vi "Configure Basic Sweep.vi"(7 "Timeout (0s)":dbl, 8 "error in (no error)":errorcluster, 9 "Repeat (T: Enable)":bool=TRUE, 10 "Pre Sweep Delay (0s)":dbl, 11 "VISA resource name":refnum<visa-resource-name>) -> (0 "error out":errorcluster, 3 "VISA resource name out":refnum<visa-resource-name>)   [LabVIEW 2014, in "Stanford Research SR1.lvlib"]
doc: "Configures the basic attributes of the Sweep."
uses:
  Stanford Research SR1.lvlib
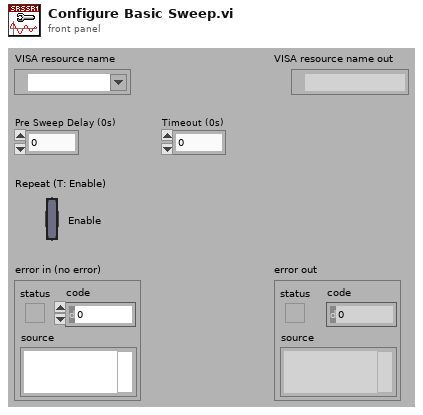
[diagram p1: front panel]
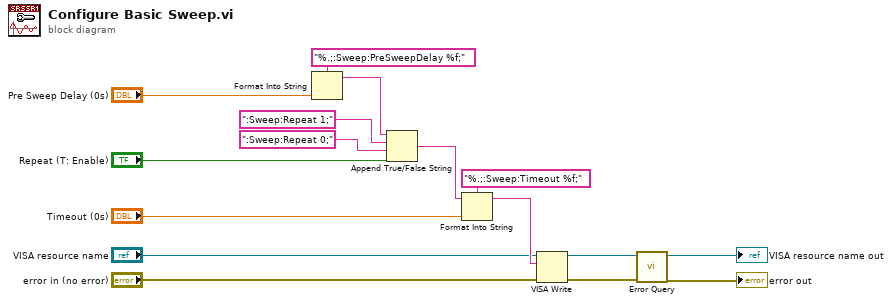
[diagram p0: block diagram]
diagram:
  n1 = Format Into String(format string="%.;:Sweep:PreSweepDelay %f;", "Pre Sweep Delay (0s)") -> (resulting string=w14:string)  [unwired: 2 in, 1 out]
  n2 = Append True/False String(1:"Repeat (T: Enable)", 2:":Sweep:Repeat 0;", 3:":Sweep:Repeat 1;", 4:w14) -> (0:w10:string)
  n3 = Format Into String(format string="%.;:Sweep:Timeout %f;", initial string=w10, "Timeout (0s)") -> (resulting string=w7:string)  [unwired: 1 in, 1 out]
  n4 = VISA Write(VISA resource name="VISA resource name", write buffer=w7, error in (no error)="error in (no error)") -> (VISA resource name out=w4:refnum<visa-resource-name>, error out=w3:errorcluster)  [unwired: 1 out]
  n5 = call "Error Query.vi"("error in (no error)"=w3, "VISA resource name"=w4) -> ("error out"=→"error out":errorcluster, "VISA resource name out"=→"VISA resource name out":refnum<visa-resource-name>)  [unwired: 6 in, 2 out]
